vi "flattenVelocityToXML.vi"   [LabVIEW 2012, in "UnitsAndXML.lvlib"]
doc: "Generates an XML string for <B>velocity</B> in the unit specified in <B>velocityUnitInXML</B>. Connect <B>velocity</B> and <B>velocityAgain</B> to the same source. The VI uses <B>velocityAgain</B> to obtain the data name."
uses:
  <userlib>/Common/UnitsAndXML/UnitsAndXML.lvlib
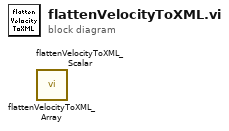
[diagram p0: block diagram]
diagram:
  n1 = call <userlib>:"flattenVelocityToXML_Array.vi"() -> ()  [unwired: 10 in, 2 out]
  n2 = call <userlib>:"flattenVelocityToXML_Scalar.vi"() -> ()  [unwired: 10 in, 2 out]
